vi "Stepper DAQ (Core).vi"(8 "error in (no error)":errorcluster, 11 "BIBA 2017 Config in":T1) -> (0 "error out":errorcluster, 2 "Axis Data":T5, 3 "BIBA 2017 Config out":T1)   [LabVIEW 2016, in "SMD-7615.lvlib"]
uses:
  SMD-7615.lvlib
  CTL/Axis Data.ctl
  CTL/Motion IO.ctl
  CTL/Digital Lines (Read).ctl
  CTL/Status.ctl
  CTL/Encoder.ctl
  CTL/Position.ctl
  CTL/Stepper Drive Config.ctl
  CTL/SV General.ctl
  CTL/SV Inputs.ctl
  CTL/SV Outputs.ctl
  <resource>/objmgr/nimcca.rc
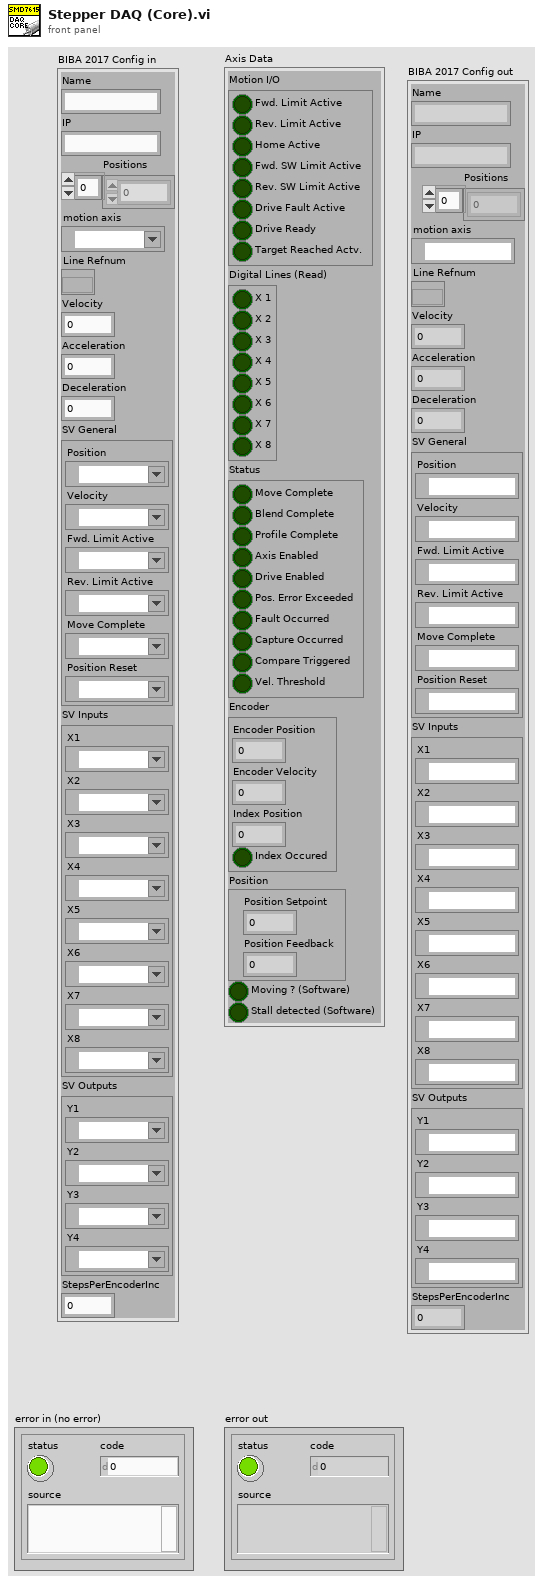
[diagram p1: front panel]
types:
  T1 = typedef "SMD-7615.lvlib/Stepper Drive Config.ctl" = cluster{"Name":string, "IP":string, "Positions":dbl[], "motion axis ":refnum<k21>, "Line Refnum":refnum<k20>, "Velocity":dbl, "Acceleration":dbl, "Deceleration":dbl, "SV General":T2, "SV Inputs":T3, "SV Outputs":T4, "StepsPerEncoderInc":i32}
  T2 = typedef "SMD-7615.lvlib/SV General.ctl" = cluster{"Position":refnum<k21>, "Velocity":refnum<k21>, "Fwd. Limit Active":refnum<k21>, "Rev. Limit Active":refnum<k21>, "Move Complete":refnum<k21>, "Position Reset":refnum<k21>}
  T3 = typedef "SMD-7615.lvlib/SV Inputs.ctl" = cluster{"X1":refnum<k21>, "X2":refnum<k21>, "X3":refnum<k21>, "X4":refnum<k21>, "X5":refnum<k21>, "X6":refnum<k21>, "X7":refnum<k21>, "X8":refnum<k21>}
  T4 = typedef "SMD-7615.lvlib/SV Outputs.ctl" = cluster{"Y1":refnum<k21>, "Y2":refnum<k21>, "Y3":refnum<k21>, "Y4":refnum<k21>}
  T5 = typedef "SMD-7615.lvlib/Axis Data.ctl" = cluster{"Motion I/O":T6, "Digital Lines (Read)":T7, "Status":T8, "Encoder":T9, "Position":T10, "Moving ? (Software)":bool, "Stall detected (Software)":bool}
  T6 = typedef "SMD-7615.lvlib/Motion IO.ctl" = cluster{"Fwd. Limit Active":bool, "Rev. Limit Active":bool, "Home Active":bool, "Fwd. SW Limit Active":bool, "Rev. SW Limit Active":bool, "Drive Fault Active":bool, "Drive Ready":bool, "Target Reached Actv.":bool}
  T7 = typedef "SMD-7615.lvlib/Digital Lines (Read).ctl" = cluster{"X 1":bool, "X 2":bool, "X 3":bool, "X 4":bool, "X 5":bool, "X 6":bool, "X 7":bool, "X 8":bool}
  T8 = typedef "SMD-7615.lvlib/Status.ctl" = cluster{"Move Complete":bool, "Blend Complete":bool, "Profile Complete":bool, "Axis Enabled":bool, "Drive Enabled":bool, "Pos. Error Exceeded":bool, "Fault Occurred":bool, "Capture Occurred":bool, "Compare Triggered":bool, "Vel. Threshold":bool}
  T9 = typedef "SMD-7615.lvlib/Encoder.ctl" = cluster{"Encoder Position":dbl, "Encoder Velocity":dbl, "Index Position":dbl, "Index Occured":bool}
  T10 = typedef "SMD-7615.lvlib/Position.ctl" = cluster{"Position Setpoint":dbl, "Position Feedback":dbl}
  T11 = cluster{"[0]":bool, "[1]":bool, "[2]":bool, "[3]":bool, "[4]":bool, "[5]":bool, "[6]":bool, "[7]":bool}
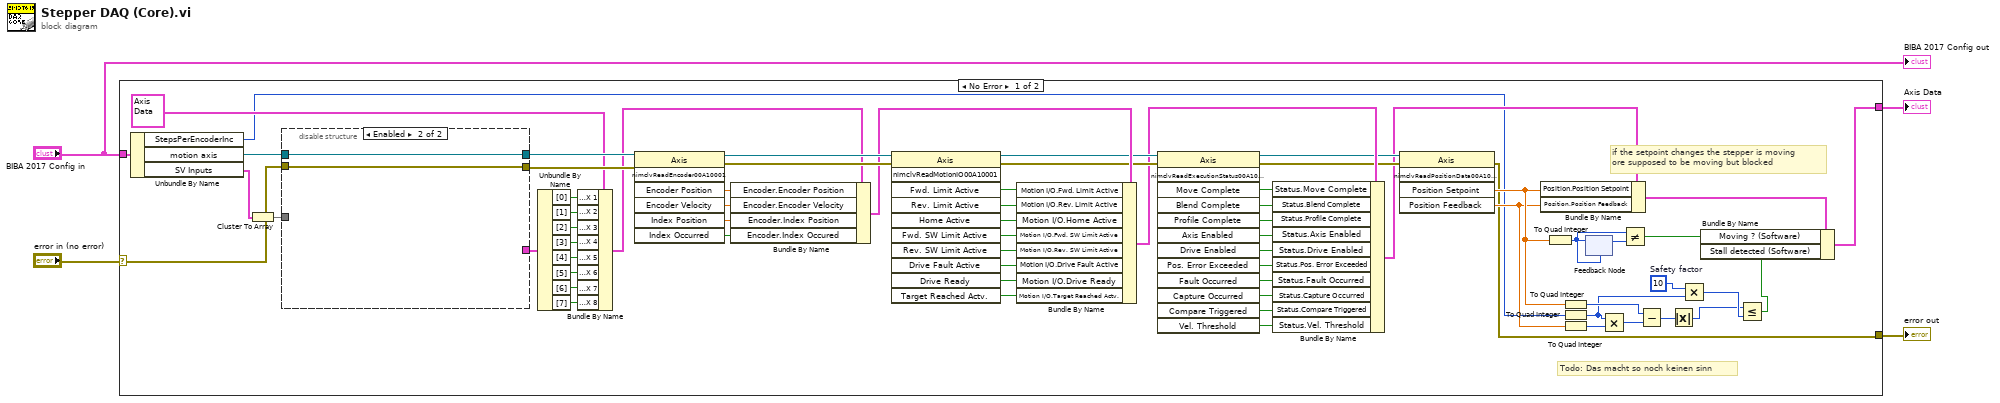
[diagram p0: block diagram]
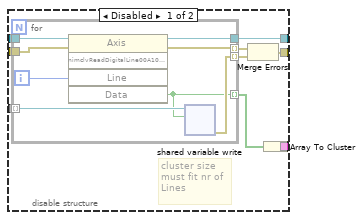
[diagram p2: hidden frame]
diagram:
  n1 = case shown="No Error" "error in (no error)" {
    selector: "error in (no error)" -> [w63 w91]
    tunnel: [w7 w91] -> w2
    tunnel: "BIBA 2017 Config in" -> [w64 _]
    tunnel: [w22 _] -> w3
    frame No Error {
      w11 = i64 10  # Safety factor
      # "Todo: Das macht so noch keinen sinn"
      # "if the setpoint changes the stepper is moving \nore supposed to be moving but blocked"
      n2 = Unbundle By Name(w64) -> ("StepsPerEncoderInc"=w6:i32, "motion axis"=w65:refnum<k21>, "SV Inputs"=w68:T3)
      n3 = Cluster To Array(cluster=w68) -> (array=w69:refnum<k21>[])
      n4 = disable-structure shown="Enabled" {
        disable-tunnel: w69 -> [w79 _]
        disable-tunnel: [w78 w89] -> w67
        disable-tunnel: [w76 w90] -> w66
        disable-tunnel: w65 -> [w75 w90]
        disable-tunnel: w63 -> [w74 w89]
        disable-tunnel: [w72 _] -> w62
        frame Disabled {
          # "cluster size\nmust fit nr of\nLines"
          n5 = for {
            tunnel: w74 -> [w87]
            tunnel: w75 -> [w88]
            tunnel: [w86] -> w76
            tunnel: [w84] -> w77 mode=indexing
            tunnel: w79 -> [w83] mode=indexing
            tunnel: [w82] -> w80 mode=indexing
            tunnel: [w81] -> w73 mode=indexing
            i -> [w85]
            n6 = invoke class="Axis" method="nimclvReadDigitalLine00A10001"(reference=w88, error in=w87, "Line"=w85) -> (reference out=w86:refnum<k21>, error out=w84:errorcluster, "Data"=w81:bool)  [unwired: 2 in, 2 out]
            n7 = shared-variable-write(w83, w81) -> (w82:errorcluster)  [unwired: 1 in, 1 out]
          }
          n8 = Merge Errors(w77, w80) -> (w78:errorcluster)
          n9 = Array To Cluster(array=w73) -> (cluster=w72:T11)
        }
        frame Enabled {
        }
      }
      n10 = Unbundle By Name(w62) -> ("[0]"=w60:bool, "[1]"=w59:bool, "[2]"=w58:bool, "[3]"=w57:bool, "[4]"=w56:bool, "[5]"=w55:bool, "[6]"=w54:bool, "[7]"=w53:bool)
      n11 = Bundle By Name(cluster=T5 {"Motion I/O"={"Fwd. Limit Active"=FALSE, "Rev. Limit Active"=FALSE, "Home Active"=FALSE, "Fwd. SW Limit Active"=FALSE, "Rev. SW Limit Active"=FALSE, "Drive Fault Active"=FALSE, "Drive Ready"=FALSE, "Target Reached Actv."=FALSE}, "Digital Lines (Read)"={"X 1"=FALSE, "X 2"=FALSE, "X 3"=FALSE, "X 4"=FALSE, "X 5"=FALSE, "X 6"=FALSE, "X 7"=FALSE, "X 8"=FALSE}, "Status"={"Move Complete"=FALSE, "Blend Complete"=FALSE, "Profile Complete"=FALSE, "Axis Enabled"=FALSE, "Drive Enabled"=FALSE, "Pos. Error Exceeded"=FALSE, "Fault Occurred"=FALSE, "Capture Occurred"=FALSE, "Compare Triggered"=FALSE, "Vel. Threshold"=FALSE}, "Encoder"={"Encoder Position"=0.0, "Encoder Velocity"=0.0, "Index Position"=0.0, "Index Occured"=FALSE}, "Position"={"Position Setpoint"=0.0, "Position Feedback"=0.0}, "Moving ? (Software)"=FALSE, "Stall detected (Software)"=FALSE} ("Axis Data"), "Digital Lines (Read).X 1"=w60, "Digital Lines (Read).X 2"=w59, "Digital Lines (Read).X 3"=w58, "Digital Lines (Read).X 4"=w57, "Digital Lines (Read).X 5"=w56, "Digital Lines (Read).X 6"=w55, "Digital Lines (Read).X 7"=w54, "Digital Lines (Read).X 8"=w53) -> (w5:T5)
      n12 = invoke class="Axis" method="nimclvReadEncoder00A10001"(reference=w66, error in=w67) -> (reference out=w70:refnum<k21>, error out=w71:errorcluster, "Encoder Position"=w52:dbl, "Encoder Velocity"=w51:dbl, "Index Position"=w50:dbl, "Index Occurred"=w49:bool)  [unwired: 5 in, 1 out]
      n13 = Bundle By Name(cluster=w5, "Encoder.Encoder Position"=w52, "Encoder.Encoder Velocity"=w51, "Encoder.Index Position"=w50, "Encoder.Index Occured"=w49) -> (w48:T5)
      n14 = invoke class="Axis" method="nimclvReadMotionIO00A10001"(reference=w70, error in=w71) -> (reference out=w39:refnum<k21>, error out=w38:errorcluster, "Fwd. Limit Active"=w47:bool, "Rev. Limit Active"=w46:bool, "Home Active"=w45:bool, "Fwd. SW Limit Active"=w44:bool, "Rev. SW Limit Active"=w43:bool, "Drive Fault Active"=w42:bool, "Drive Ready"=w41:bool, "Target Reached Actv."=w40:bool)  [unwired: 9 in, 1 out]
      n15 = Bundle By Name(cluster=w48, "Motion I/O.Fwd. Limit Active"=w47, "Motion I/O.Rev. Limit Active"=w46, "Motion I/O.Home Active"=w45, "Motion I/O.Fwd. SW Limit Active"=w44, "Motion I/O.Rev. SW Limit Active"=w43, "Motion I/O.Drive Fault Active"=w42, "Motion I/O.Drive Ready"=w41, "Motion I/O.Target Reached Actv."=w40) -> (w37:T5)
      n16 = invoke class="Axis" method="nimclvReadExecutionStatus00A10001"(reference=w39, error in=w38) -> (reference out=w25:refnum<k21>, error out=w26:errorcluster, "Move Complete"=w27:bool, "Blend Complete"=w28:bool, "Profile Complete"=w29:bool, "Axis Enabled"=w30:bool, "Drive Enabled"=w31:bool, "Pos. Error Exceeded"=w32:bool, "Fault Occurred"=w33:bool, "Capture Occurred"=w34:bool, "Compare Triggered"=w35:bool, "Vel. Threshold"=w36:bool)  [unwired: 11 in, 1 out]
      n17 = Bundle By Name(cluster=w37, "Status.Move Complete"=w27, "Status.Blend Complete"=w28, "Status.Profile Complete"=w29, "Status.Axis Enabled"=w30, "Status.Drive Enabled"=w31, "Status.Pos. Error Exceeded"=w32, "Status.Fault Occurred"=w33, "Status.Capture Occurred"=w34, "Status.Compare Triggered"=w35, "Status.Vel. Threshold"=w36) -> (w24:T5)
      n18 = invoke class="Axis" method="nimclvReadPositionData00A10001"(reference=w25, error in=w26) -> (error out=w7:errorcluster, "Position Setpoint"=w18:dbl, "Position Feedback"=w17:dbl)  [unwired: 3 in, 2 out]
      n19 = Bundle By Name(cluster=w24, "Position.Position Setpoint"=w18, "Position.Position Feedback"=w17) -> (w23:T5)
      n20 = To Quad Integer(1:w18) -> (0:w21:i64)
      n21 = To Quad Integer(1:w18) -> (0:w13:i64)
      n22 = To Quad Integer(1:w6) -> (0:w10:i64)
      n23 = To Quad Integer(1:w17) -> (0:w16:i64)
      n24 = feedback-in #1(w21) -> ()
      n25 = feedback #1(w21) -> (w19:i64)
      n26 = Multiply(x=w10, y=w16) -> (x*y=w15:i64)
      n27 = Not Equal?(x=w21, y=w19) -> (x != y?=w20:bool)
      n28 = Subtract(x=w13, y=w15) -> (x-y=w14:i64)
      n29 = Absolute Value(x=w14) -> (abs(x)=w8:i64)
      n30 = Multiply(x=w11, y=w10) -> (x*y=w9:i64)
      n31 = Less Or Equal?(x=w8, y=w9) -> (x <= y?=w12:bool)
      n32 = Bundle By Name(cluster=w23, "Moving ? (Software)"=w20, "Stall detected (Software)"=w12) -> (w22:T5)
    }
    frame Error {
    }
  }
  "Axis Data" <- w3
  "error out" <- w2
  "BIBA 2017 Config out" <- "BIBA 2017 Config in"
